vi "LinxDigitalWrite.vi"(8 "Error In":errorcluster, 9 "Values":bool[](array[boolean]), 10 "Channels":u8[](array[numeric]), 11 "LINX Resource":T1) -> (0 "Error Out":errorcluster, 3 "LINX Resource":T1)   [LabVIEW 2014, in "LMH-LINX.lvlib" / "Local IO.lvlib"]
uses:
  Local IO.lvlib
  Type Defs/LINX Ref.ctl
  Type Defs/Platform.ctl
  Type Defs/Interface.ctl
  Device/Type Defs/LINX Device Config.ctl
  Device/Type Defs/TCP Config.ctl
  Device/Type Defs/Channels.ctl
  <vilib>/myRIO/Instrument Drivers/Onboard IO/DIO/DIO.lvlib
  myRIO/myRIO.lvlib
  liblinxdevice.dll
  LMH-LINX.lvlib
  Device/Device.lvlib
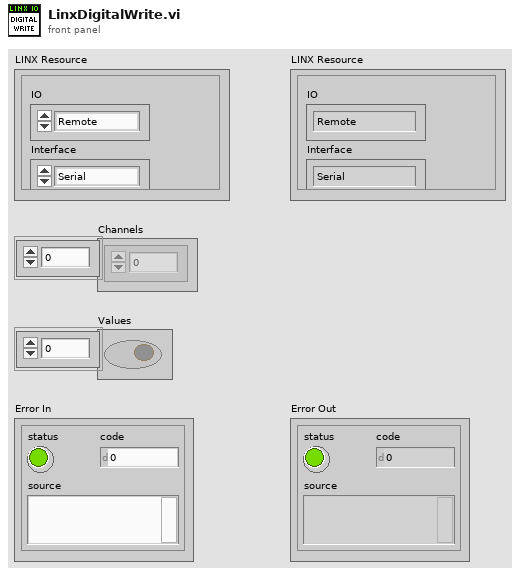
[diagram p1: front panel]
types:
  T1 = typedef "LMH-LINX.lvlib/LINX Ref.ctl" = cluster{"IO":T2, "Interface":T3, "LINX Device Config":T4}
  T2 = typedef "LMH-LINX.lvlib/Platform.ctl" = enum16{"Remote", "Local"}
  T3 = typedef "LMH-LINX.lvlib/Interface.ctl" = enum16{"Serial", "TCP"}
  T4 = typedef "LMH-LINX.lvlib/Device.lvlib/LINX Device Config.ctl" = cluster{"Interface":T3, "COM Port":refnum<visa-resource-name>, "TCP Configuration":T5, "Device Family":u8, "Device ID":u8, "Device Name":string, "TCP Ref":refnum<k5>, "Channels":T6}
  T5 = typedef "LMH-LINX.lvlib/Device.lvlib/TCP Config.ctl" = cluster{"IP Address":string, "Port":u16}
  T6 = typedef "LMH-LINX.lvlib/Channels.ctl" = cluster{"DI":u8[], "DO":u8[], "AI":u8[], "AO":u8[], "PWM":u8[], "QE":u8[], "UART":u8[], "I2C 2":u8[], "SPI":u8[], "CAN":u8[], "Servo":u8[], "AI Ref (V)":dbl, "AI Resolution (Bits)":u8, "AO Ref (V)":dbl, "AO Resolution (Bits)":u8}
  T7 = typedef "DIO.lvlib/DIO Reference.ctl" = cluster{"myRIO Reference":T8, "DIO Channels List":T12}
  T8 = typedef "myRIO Generic Hardware Reference.ctl" = cluster{"myRIO Model":T9, "myRIO Hardware Reference":T10}
  T9 = typedef "Hardware Version Enum.ctl" = enum16{"Unknown", "myRIO-1900", "myRIO-1950"}
  T10 = typedef "myRIO v1.0 Reference.ctl" = cluster{"Generic FPGA Reference":T11, "Allow multiple opens":bool}
  T11 = typedef "Generic FPGA Reference.ctl" = refnum<k20>
  T12 = typedef "DIO Channels List.ctl" = T13[]
  T13 = typedef "DIO Channels Enum.ctl" = enum16{"Not Connected", "C/DIO0", "C/DIO1", "C/DIO2", "C/DIO3", "C/DIO4", "C/DIO5", "C/DIO6", "C/DIO7", "A/DIO0", "A/DIO1", "A/DIO2", "A/DIO3", "A/DIO4", "A/DIO5", "A/DIO6", "A/DIO7", "A/DIO8", "A/DIO9", "A/DIO10", "A/DIO11", "A/DIO12", "A/DIO13", "A/DIO14", "A/DIO15", "B/DIO0", "B/DIO1", "B/DIO2", "B/DIO3", "B/DIO4", "B/DIO5", "B/DIO6", "B/DIO7", "B/DIO8", "B/DIO9", "B/DIO10", "B/DIO11", "B/DIO12", "B/DIO13", "B/DIO14", "B/DIO15", "LED0", "LED1", "LED2", "LED3", "Button0"}
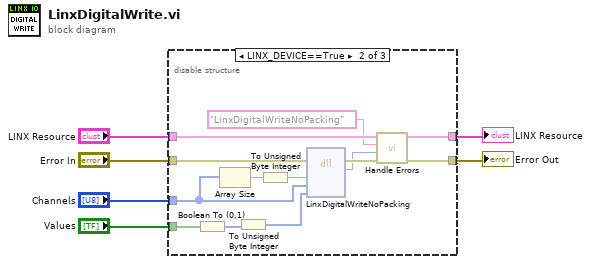
[diagram p0: block diagram]
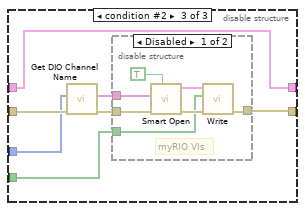
[diagram p3: hidden frame]
diagram:
  n1 = disable-structure shown="LINX_DEVICE==True" {
    disable-tunnel: "LINX Resource" -> [w8 w11 w24]
    disable-tunnel: "Error In" -> [w7 w21 w26]
    disable-tunnel: [w7 w13 w25] -> w4
    disable-tunnel: [w8 w12 w24] -> w3
    disable-tunnel: "Channels" -> [_ w18 w23]
    disable-tunnel: "Values" -> [_ w17 w22]
    frame condition #0 (active) {
    }
    frame condition #1 {
      n2 = Boolean To (0,1)(Boolean=w17) -> (0, 1=w16:i16[])
      n3 = Array Size(array=w18) -> (size(s)=w20:i32)
      n4 = To Unsigned Byte Integer(number=w16) -> (unsigned 8bit integer=w15:u8[])
      n5 = To Unsigned Byte Integer(number=w20) -> (unsigned 8bit integer=w19:u8)
      n6 = dll-call lib="liblinxdevice.*" fn="LinxDigitalWriteNoPacking"(error in=w21, "numChans"=w19, "channels"=w18, "values"=w15) -> (error out=w14:errorcluster, "LinxStatus"=w9:i32)  [unwired: 5 in, 1 out]
      n7 = call <vilib>:"Handle Errors.vi"("Error In"=w14, "LinxStatus"=w9, "Function Name"="LinxDigitalWriteNoPacking", "LINX Resource"=w11) -> ("Error Out"=w13:errorcluster, "LINX Resource"=w12:T1)  [unwired: 6 in]
    }
    frame condition #2 {
      n8 = call "Get DIO Channel Name.vi"("Error In"=w26, "DIO Channel Nums"=w23) -> ("Error Out"=w27:errorcluster, "DIO Channels"=w28:string[])  [unwired: 8 in]
      n9 = disable-structure shown="Disabled" {
        disable-tunnel: w28 -> [w32 _]
        disable-tunnel: w27 -> [w33 w36]
        disable-tunnel: [w35 w36] -> w25
        disable-tunnel: w22 -> [w29 _]
        frame Disabled {
          # "myRIO VIs"
          n10 = call <vilib>:"Smart Open.vi"("Allow multiple opens?"=TRUE, "error in (no error)"=w33, "Channel Names"=w32) -> ("error out"=w34:errorcluster, "DIO Ref Out"=w31:T7)  [unwired: 7 in]
          n11 = call <vilib>:"Write.vi"("error in (no error)"=w34, "Values"=w29, "DIO Ref In"=w31) -> ("error out"=w35:errorcluster)  [unwired: 6 in, 1 out]
        }
        frame Enabled {
          # "myRIO Support Disabled"
        }
      }
    }
  }
  "Error Out" <- w4
  "LINX Resource" <- w3
